vi "Query PC Beamage Version.vi"(8 "error in":errorcluster) -> (0 "error out":errorcluster, 2 "PC Beamage Version":string)   [LabVIEW 2009]
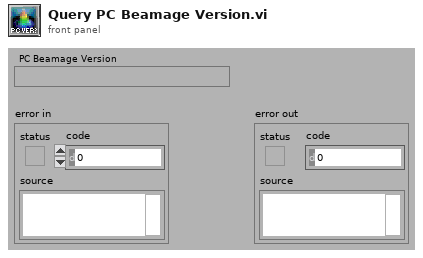
[diagram p1: front panel]
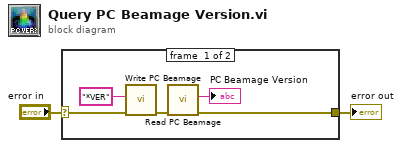
[diagram p0: block diagram]
diagram:
  n1 = case shown="No Error" "error in" {
    selector: "error in" -> [w5 w8]
    tunnel: [w4 w8] -> w1
    frame #0 {
      n2 = call "Write PC Beamage.vi"("error in"=w5, "command"="*VER") -> ("error out"=w3:errorcluster)  [unwired: 9 in]
      n3 = call "Read PC Beamage.vi"("error in"=w3) -> ("error out"=w4:errorcluster, "Reply"=→"PC Beamage Version":string)  [unwired: 9 in]
    }
    frame #1 {
    }
  }
  "error out" <- w1
